vi "Open FITS Reference.vi"(8 "error in (no error)":errorcluster, 11 "Save Image in":refnum<class "Save Image.lvclass">) -> (0 "error out":errorcluster, 3 "Save Image out":refnum<class "Save Image.lvclass">)   [LabVIEW 2018, in "Save Image.lvclass"]
uses:
  Save Image.lvclass
  <userlib>/gfitsio/cfitsio-bitpix.ctl
  Save Image.lvclass/Save Image.ctl
  <userlib>/gfitsio/gfitsio.lvlib
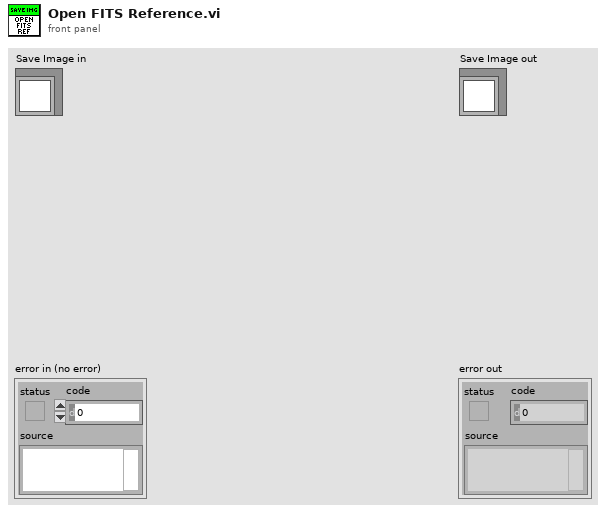
[diagram p1: front panel]
types:
  T1 = enum16{"open", "open or create", "create or replace", "create", "open (read only)"}
  T2 = enum16{"open", "open or create", "create", "create or replace"}
  T3 = typedef "gfitsio.lvlib/cfitsio-bitpix.ctl" = i32
  T4 = typedef "gfitsio.lvlib/gfitsio-refnum.ctl" = refnum<k1>
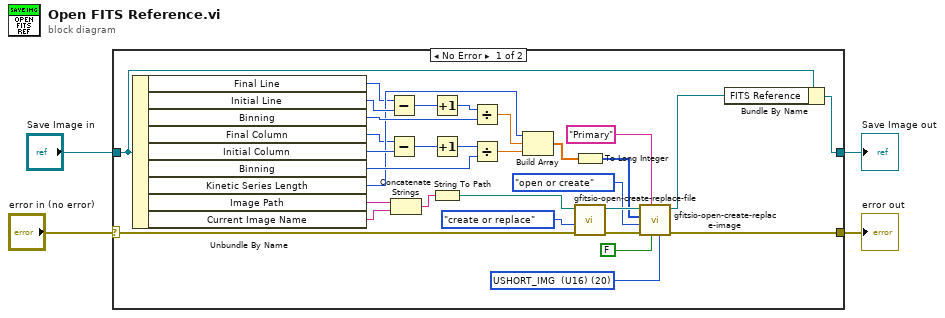
[diagram p0: block diagram]
diagram:
  n1 = case shown="No Error" "error in (no error)" {
    selector: "error in (no error)" -> [w11 w37]
    tunnel: [w6 w37] -> w3
    tunnel: [w7 w36] -> w1
    tunnel: "Save Image in" -> [w8 w36]
    frame No Error {
      w31 = T3 20 items=["<invalid type>"=0, "BYTE_IMG  (U8)"=8, "SHORT_IMG  (I16)"=16, "USHORT_IMG  (U16)"=20, "LONG_IMG  (I32)"=32, "ULONG_IMG  (U32)"=40, "FLOAT_IMG  (SGL)"=-32, "DOUBLE_IMG  (DBL)"=-64] ("image data type")
      n2 = Unbundle By Name(w8) -> ("Final Line"=w18:u16, "Initial Line"=w23:u16, "Binning"=w24:u16, "Final Column"=w17:u16, "Initial Column"=w25:u16, "Binning"=w26:u16, "Kinetic Series Length"=w19:u16, "Image Path"=w16:string, "Current Image Name"=w20:string)
      n3 = Subtract(x=w18, y=w23) -> (x-y=w21:u16)
      n4 = Subtract(x=w17, y=w25) -> (x-y=w22:u16)
      n5 = Concatenate Strings(w16, w20) -> (w30:string)
      n6 = Increment(x=w21) -> (x+1=w15:u16)
      n7 = Increment(x=w22) -> (x+1=w14:u16)
      n8 = String To Path(string=w30) -> (path=w29:path)
      n9 = Divide(x=w15, y=w24) -> (x/y=w13:dbl)
      n10 = Divide(x=w14, y=w26) -> (x/y=w12:dbl)
      n11 = Build Array(w19, w13, w12) -> (w10:dbl[])
      n12 = To Long Integer(number=w10) -> (32bit integer=w9:i32[])
      n13 = call <userlib>:"gfitsio-open-create-replace-file.vi"("error in (no error)"=w11, "function (open)"=T1."create or replace", "file path (dialog if empty)"=w29) -> ("error out"=w35:errorcluster, "gfits refnum"=w34:T4)  [unwired: 6 in, 1 out]
      n14 = call <userlib>:"gfitsio-open-create-replace-image.vi"("image data type"=w31, "advisory dialog? (display:T)"=FALSE, "hdu name (dialog if empty)"="Primary" ("prompt"), "error in (no error)"=w35, "function (create or replace)"=T2."open or create" ("function (open or create)"), "naxes"=w9, "gfits refnum"=w34) -> ("error out"=w6:errorcluster, "dup gfits refnum"=w5:T4)  [unwired: 2 in, 1 out]
      n15 = Bundle By Name(cluster=w8, "FITS Reference"=w5) -> (w7:refnum<class "Save Image.lvclass">)
    }
    frame Error {
    }
  }
  "error out" <- w3
  "Save Image out" <- w1
